vi "FGV用法_DataFGV.vi"() -> ()   [LabVIEW 2015]
panel:
  out "data":cluster{string, i32}
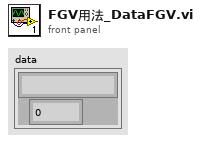
[diagram p1: front panel]
types:
  T1 = typedef "Action_Data.ctl" = enum16{"Initialize", "Get Data", "Set Data", "Delete Data", "Idle"}
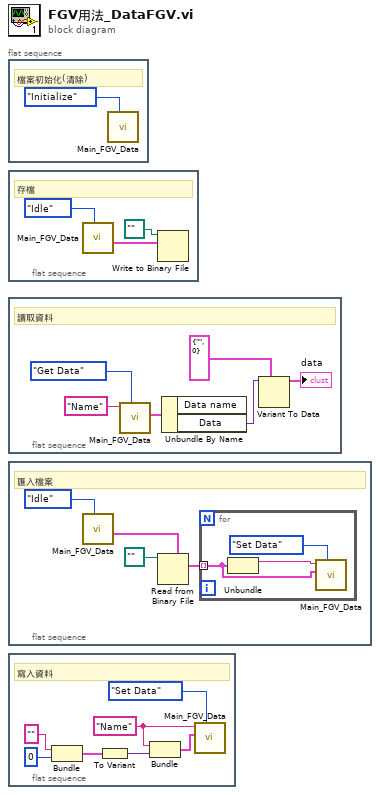
[diagram p0: block diagram]
diagram:
  n1 = flat-sequence {
    frame #0 {
      # "檔案初始化(清除)"
      n2 = call "Main_FGV_Data.vi"("Action_Data"=Action_Data."Initialize") -> ()  [unwired: 9 in, 2 out]
    }
  }
  n3 = flat-sequence {
    frame #0 {
      # "存檔"
      n4 = call "Main_FGV_Data.vi"("Action_Data"=Action_Data."Idle") -> ("Data Array out"=w3:cluster{"Data name":string, "Data":variant}[])  [unwired: 9 in, 1 out]
      n5 = Write to Binary File(file (use dialog)=path "", data=w3) -> ()  [unwired: 4 in, 3 out]
    }
  }
  n6 = flat-sequence {
    frame #0 {
      # "讀取資料"
      n7 = call "Main_FGV_Data.vi"("Action_Data"=Action_Data."Get Data", "Data name"="Name") -> ("Data  Out"=w8:cluster{"Data name":string, "Data":variant})  [unwired: 8 in, 1 out]
      n8 = Unbundle By Name(w8) -> ("Data"=w7:variant)  [unwired: 1 out]
      n9 = Variant To Data(type=cluster{string, i32} {"", 0} ("dataForm"), Variant=w7) -> (data=→"data":cluster{string, i32})  [unwired: 1 in, 1 out]
    }
  }
  n10 = flat-sequence {
    frame #0 {
      # "匯入檔案"
      n11 = call "Main_FGV_Data.vi"("Action_Data"=Action_Data."Idle") -> ("Data Array out"=w11:cluster{"Data name":string, "Data":variant}[])  [unwired: 9 in, 1 out]
      n12 = Read from Binary File(5:w11, 11:path "" ("file (use dialog)")) -> (2:w13:cluster{"Data name":string, "Data":variant}[])  [unwired: 4 in, 3 out]
      n13 = for {
        tunnel: w13 -> [w15] mode=indexing
        n14 = Unbundle(w15) -> ("Data name"=w16:string)  [unwired: 1 out]
        n15 = call "Main_FGV_Data.vi"("Action_Data"=Action_Data."Set Data", "Data In"=w15, "Data name"=w16) -> ()  [unwired: 7 in, 2 out]
      }
    }
  }
  n16 = flat-sequence {
    frame #0 {
      w19 = "Name" ("Data name")
      # "寫入資料"
      n17 = Bundle("", 0) -> (w23:cluster{string, i32})  [unwired: 1 in]
      n18 = To Variant(anything=w23) -> (Variant=w20:variant)
      n19 = Bundle("Data name"=w19, "Variant"=w20) -> (w18:cluster{"Data name":string, "Variant":variant})  [unwired: 1 in]
      n20 = call "Main_FGV_Data.vi"("Action_Data"=Action_Data."Set Data", "Data In"=w18, "Data name"=w19) -> ()  [unwired: 7 in, 2 out]
    }
  }
